vi "Shock&Dyanamics Laboratory - DROPBEAR_June2022_Rev3.vi"() -> ()   [LabVIEW 2019] (continued)
  T49 = cluster{"Voltage Max Ch0":dbl, "Voltage Max Ch 1":dbl, "Voltage Max Ch 2":dbl, "Voltage Max Ch 3":dbl, "Voltage Max Ch 4":dbl, "Voltage Max Ch 5":dbl, "Voltage Max  Ch 6":dbl, "Voltage Max Ch 7":dbl, "Voltage Max Ch 8":dbl, "Voltage Max Ch 9":dbl, "Voltage Max Ch 10":dbl, "Voltage Max Ch 11":dbl, "Voltage Max Ch 12":dbl, "Voltage Max Ch 13":dbl, "Voltage Max Ch 14":dbl, "Voltage Max Ch 15":dbl, "Voltage Max Ch 16":dbl, "Voltage Max Ch 17":dbl, "Voltage Max Ch 18":dbl, "Voltage Max Ch 19":dbl, "Voltage Max Ch 20":dbl, "Voltage Max Ch 21":dbl, "Voltage Max Ch 22":dbl, "Voltage Max Ch 23":dbl, "Voltage Max Ch 24":dbl, "Voltage Max  Ch 7":dbl, "Voltage Max Ch 6":dbl, "Voltage Max Ch 25":dbl, "Voltage Max Ch 26":dbl, "Voltage Max Ch 27":dbl, "Voltage Max Ch 28":dbl, "Voltage Max Ch0 2":dbl}
  T50 = cluster{"Sensitivity 0":dbl, "Sensitivity 1":dbl, "Sensitivity 2":dbl, "Sensitivity 3":dbl, "Sensitivity 4":dbl, "Sensitivity 5":dbl, "Sensitivity 6":dbl, "Sensitivity 7":dbl, "Sensitivity 8":dbl, "Sensitivity 9":dbl, "Sensitivity 10":dbl, "Sensitivity 11":dbl, "Sensitivity 12":dbl, "Sensitivity 13":dbl, "Sensitivity 14":dbl, "Sensitivity 15":dbl, "Sensitivity 16":dbl, "Sensitivity 17":dbl, "Sensitivity 18":dbl, "Sensitivity 19":dbl, "Sensitivity 20":dbl, "Sensitivity 21":dbl, "Sensitivity 22":dbl, "Sensitivity 23":dbl, "Sensitivity 24":dbl, "Sensitivity 25":dbl, "Sensitivity 26":dbl, "Sensitivity 27":dbl, "Sensitivity 28":dbl, "Sensitivity 29":dbl, "Sensitivity 30":dbl, "Sensitivity 31":dbl}
  T51 = cluster{"Sens Fac 0":enum16{"uV/MU", "mV/MU", "V/MU"}, "Sens Fac 1":enum16{"uV/MU", "mV/MU", "V/MU"}, "Sens Fac 2":enum16{"uV/MU", "mV/MU", "V/MU"}, "Sens Fac 3":enum16{"uV/MU", "mV/MU", "V/MU"}, "Sens Fac 4":enum16{"uV/MU", "mV/MU", "V/MU"}, "Sens Fac 5":enum16{"uV/MU", "mV/MU", "V/MU"}, "Sens Fac 6":enum16{"uV/MU", "mV/MU", "V/MU"}, "Sens Fac 7":enum16{"uV/MU", "mV/MU", "V/MU"}, "Sens Fac 8":enum16{"uV/MU", "mV/MU", "V/MU"}, "Sens Fac 9":enum16{"uV/MU", "mV/MU", "V/MU"}, "Sens Fac 10":enum16{"uV/MU", "mV/MU", "V/MU"}, "Sens Fac 11":enum16{"uV/MU", "mV/MU", "V/MU"}, "Sens Fac 12":enum16{"uV/MU", "mV/MU", "V/MU"}, "Sens Fac 13":enum16{"uV/MU", "mV/MU", "V/MU"}, "Sens Fac 14":enum16{"uV/MU", "mV/MU", "V/MU"}, "Sens Fac 15":enum16{"uV/MU", "mV/MU", "V/MU"}, "Sens Fac 16":enum16{"uV/MU", "mV/MU", "V/MU"}, "Sens Fac 17":enum16{"uV/MU", "mV/MU", "V/MU"}, "Sens Fac 18":enum16{"uV/MU", "mV/MU", "V/MU"}, "Sens Fac 19":enum16{"uV/MU", "mV/MU", "V/MU"}, "Sens Fac 20":enum16{"uV/MU", "mV/MU", "V/MU"}, "Sens Fac 21":enum16{"uV/MU", "mV/MU", "V/MU"}, "Sens Fac 22":enum16{"uV/MU", "mV/MU", "V/MU"}, "Sens Fac 23":enum16{"uV/MU", "mV/MU", "V/MU"}, "Sens Fac 24":enum16{"uV/MU", "mV/MU", "V/MU"}, "Sens Fac 25":enum16{"uV/MU", "mV/MU", "V/MU"}, "Sens Fac 26":enum16{"uV/MU", "mV/MU", "V/MU"}, "Sens Fac 27":enum16{"uV/MU", "mV/MU", "V/MU"}, "Sens Fac 28":enum16{"uV/MU", "mV/MU", "V/MU"}, "Sens Fac 29":enum16{"uV/MU", "mV/MU", "V/MU"}, "Sens Fac 30":enum16{"uV/MU", "mV/MU", "V/MU"}, "Sens Fac 31":enum16{"uV/MU", "mV/MU", "V/MU"}}
  T52 = cluster{"SG Pair 0":bool, "SG Pair 1":bool, "SG Pair 2":bool, "SG Pair 3":bool, "SG Pair 4":bool, "SG Pair 5":bool, "SG Pair 6":bool, "SG Pair 7":bool, "SG Pair 8":bool, "SG Pair 9":bool, "SG Pair 10":bool, "SG Pair 11":bool, "SG Pair 12":bool, "SG Pair 13":bool, "SG Pair 14":bool, "SG Pair 15":bool, "SG Pair 16":bool, "SG Pair 17":bool, "SG Pair 18":bool, "SG Pair 19":bool, "SG Pair 20":bool, "SG Pair 21":bool, "SG Pair 22":bool, "SG Pair 23":bool, "SG Pair 24":bool, "SG Pair 25":bool, "SG Pair 26":bool, "SG Pair 27":bool, "SG Pair 28":bool, "SG Pair 29":bool, "SG Pair 30":bool, "SG Pair 31":bool}
  T53 = cluster{"SG Pair Ch 0":enum16{"", "Ch 1", "Ch 2", "Ch 3", "Ch 4", "Ch 5", "Ch 6", "Ch 7", "Ch 8", "Ch 9", "Ch 10", "Ch 11", "Ch 12", "Ch 13", "Ch 14", "Ch 15", "Ch 16", "Ch 17", "Ch 18", "Ch 19", "Ch 20", "Ch 21", "Ch 22", "Ch 23", "Ch 24", "Ch 25", "Ch 26", "Ch 27", "Ch 28", "Ch 29", "Ch 30", "Ch 31", "Paired", "Unpaired"}, "SG Pair Ch 1":enum16{"Ch 0", "", "Ch 2", "Ch 3", "Ch 4", "Ch 5", "Ch 6", "Ch 7", "Ch 8", "Ch 9", "Ch 10", "Ch 11", "Ch 12", "Ch 13", "Ch 14", "Ch 15", "Ch 16", "Ch 17", "Ch 18", "Ch 19", "Ch 20", "Ch 21", "Ch 22", "Ch 23", "Ch 24", "Ch 25", "Ch 26", "Ch 27", "Ch 28", "Ch 29", "Ch 30", "Ch 31", "Paired", "Unpaired"}, "SG Pair Ch 2":enum16{"Ch0", "Ch 1", "", "Ch 3", "Ch 4", "Ch 5", "Ch 6", "Ch 7", "Ch 8", "Ch 9", "Ch 10", "Ch 11", "Ch 12", "Ch 13", "Ch 14", "Ch 15", "Ch 16", "Ch 17", "Ch 18", "Ch 19", "Ch 20", "Ch 21", "Ch 22", "Ch 23", "Ch 24", "Ch 25", "Ch 26", "Ch 27", "Ch 28", "Ch 29", "Ch 30", "Ch 31", "Paired", "Unpaired"}, "SG Pair Ch 3":enum16{"Ch 0", "Ch 1", "Ch 2", "", "Ch 4", "Ch 5", "Ch 6", "Ch 7", "Ch 8", "Ch 9", "Ch 10", "Ch 11", "Ch 12", "Ch 13", "Ch 14", "Ch 15", "Ch 16", "Ch 17", "Ch 18", "Ch 19", "Ch 20", "Ch 21", "Ch 22", "Ch 23", "Ch 24", "Ch 25", "Ch 26", "Ch 27", "Ch 28", "Ch 29", "Ch 30", "Ch 31", "Paired", "Unpaired"}, "SG Pair Ch 4":enum16{"Ch 0", "Ch 1", "Ch 2", "Ch 3", "", "Ch 5", "Ch 6", "Ch 7", "Ch 8", "Ch 9", "Ch 10", "Ch 11", "Ch 12", "Ch 13", "Ch 14", "Ch 15", "Ch 16", "Ch 17", "Ch 18", "Ch 19", "Ch 20", "Ch 21", "Ch 22", "Ch 23", "Ch 24", "Ch 25", "Ch 26", "Ch 27", "Ch 28", "Ch 29", "Ch 30", "Ch 31", "Paired", "Unpaired"}, "SG Pair Ch 5":enum16{"Ch 0", "Ch 1", "Ch 2", "Ch 3", "Ch 4", "", "Ch 6", "Ch 7", "Ch 8", "Ch 9", "Ch 10", "Ch 11", "Ch 12", "Ch 13", "Ch 14", "Ch 15", "Ch 16", "Ch 17", "Ch 18", "Ch 19", "Ch 20", "Ch 21", "Ch 22", "Ch 23", "Ch 24", "Ch 25", "Ch 26", "Ch 27", "Ch 28", "Ch 29", "Ch 30", "Ch 31", "Paired", "Unpaired"}, "SG Pair Ch 6":enum16{"Ch 0", "Ch 1", "Ch 2", "Ch 3", "Ch 4", "Ch 5", "", "Ch 7", "Ch 8", "Ch 9", "Ch 10", "Ch 11", "Ch 12", "Ch 13", "Ch 14", "Ch 15", "Ch 16", "Ch 17", "Ch 18", "Ch 19", "Ch 20", "Ch 21", "Ch 22", "Ch 23", "Ch 24", "Ch 25", "Ch 26", "Ch 27", "Ch 28", "Ch 29", "Ch 30", "Ch 31", "Paired", "Unpaired"}, "SG Pair Ch 7":enum16{"Ch 0", "Ch 1", "Ch 2", "Ch 3", "Ch 4", "Ch 5", "Ch 6", "", "Ch 8", "Ch 9", "Ch 10", "Ch 11", "Ch 12", "Ch 13", "Ch 14", "Ch 15", "Ch 16", "Ch 17", "Ch 18", "Ch 19", "Ch 20", "Ch 21", "Ch 22", "Ch 23", "Ch 24", "Ch 25", "Ch 26", "Ch 27", "Ch 28", "Ch 29", "Ch 30", "Ch 31", "Paired", "Unpaired"}, "SG Pair Ch 8":enum16{"Ch 0", "Ch 1", "Ch 2", "Ch 3", "Ch 4", "Ch 5", "Ch 6", "Ch 7", "", "Ch 9", "Ch 10", "Ch 11", "Ch 12", "Ch 13", "Ch 14", "Ch 15", "Ch 16", "Ch 17", "Ch 18", "Ch 19", "Ch 20", "Ch 21", "Ch 22", "Ch 23", "Ch 24", "Ch 25", "Ch 26", "Ch 27", "Ch 28", "Ch 29", "Ch 30", "Ch 31", "Paired", "Unpaired"}, "SG Pair Ch 9":enum16{"Ch 0", "Ch 1", "Ch 2", "Ch 3", "Ch 4", "Ch 5", "Ch 6", "Ch 7", "Ch 8", "", "Ch 10", "Ch 11", "Ch 12", "Ch 13", "Ch 14", "Ch 15", "Ch 16", "Ch 17", "Ch 18", "Ch 19", "Ch 20", "Ch 21", "Ch 22", "Ch 23", "Ch 24", "Ch 25", "Ch 26", "Ch 27", "Ch 28", "Ch 29", "Ch 30", "Ch 31", "Paired", "Unpaired"}, "SG Pair Ch 10":enum16{"Ch 0", "Ch 1", "Ch 2", "Ch 3", "Ch 4", "Ch 5", "Ch 6", "Ch 7", "Ch 8", "Ch 9", "", "Ch 11", "Ch 12", "Ch 13", "Ch 14", "Ch 15", "Ch 16", "Ch 17", "Ch 18", "Ch 19", "Ch 20", "Ch 21", "Ch 22", "Ch 23", "Ch 24", "Ch 25", "Ch 26", "Ch 27", "Ch 28", "Ch 29", "Ch 30", "Ch 31", "Paired", "Unpaired"}, "SG Pair Ch 11":enum16{"Ch 0", "Ch 1", "Ch 2", "Ch 3", "Ch 4", "Ch 5", "Ch 6", "Ch 7", "Ch 8", "Ch 9", "Ch 10", "", "Ch 12", "Ch 13", "Ch 14", "Ch 15", "Ch 16", "Ch 17", "Ch 18", "Ch 19", "Ch 20", "Ch 21", "Ch 22", "Ch 23", "Ch 24", "Ch 25", "Ch 26", "Ch 27", "Ch 28", "Ch 29", "Ch 30", "Ch 31", "Paired", "Unpaired"}, "SG Pair Ch 12":enum16{"Ch 0", "Ch 1", "Ch 2", "Ch 3", "Ch 4", "Ch 5", "Ch 6", "Ch 7", "Ch 8", "Ch 9", "Ch 10", "Ch 11", "", "Ch 13", "Ch 14", "Ch 15", "Ch 16", "Ch 17", "Ch 18", "Ch 19", "Ch 20", "Ch 21", "Ch 22", "Ch 23", "Ch 24", "Ch 25", "Ch 26", "Ch 27", "Ch 28", "Ch 29", "Ch 30", "Ch 31", "Paired", "Unpaired"}, "SG Pair Ch 13":enum16{"Ch 0", "Ch 1", "Ch 2", "Ch 3", "Ch 4", "Ch 5", "Ch 6", "Ch 7", "Ch 8", "Ch 9", "Ch 10", "Ch 11", "Ch 12", "", "Ch 14", "Ch 15", "Ch 16", "Ch 17", "Ch 18", "Ch 19", "Ch 20", "Ch 21", "Ch 22", "Ch 23", "Ch 24", "Ch 25", "Ch 26", "Ch 27", "Ch 28", "Ch 29", "Ch 30", "Ch 31", "Paired", "Unpaired"}, "SG Pair Ch 14":enum16{"Ch 0", "Ch 1", "Ch 2", "Ch 3", "Ch 4", "Ch 5", "Ch 6", "Ch 7", "Ch 8", "Ch 9", "Ch 10", "Ch 11", "Ch 12", "Ch 13", "", "Ch 15", "Ch 16", "Ch 17", "Ch 18", "Ch 19", "Ch 20", "Ch 21", "Ch 22", "Ch 23", "Ch 24", "Ch 25", "Ch 26", "Ch 27", "Ch 28", "Ch 29", "Ch 30", "Ch 31", "Paired", "Unpaired"}, "SG Pair Ch 15":enum16{"Ch 0", "Ch 1", "Ch 2", "Ch 3", "Ch 4", "Ch 5", "Ch 6", "Ch 7", "Ch 8", "Ch 9", "Ch 10", "Ch 11", "Ch 12", "Ch 13", "Ch 14", "", "Ch 16", "Ch 17", "Ch 18", "Ch 19", "Ch 20", "Ch 21", "Ch 22", "Ch 23", "Ch 24", "Ch 25", "Ch 26", "Ch 27", "Ch 28", "Ch 29", "Ch 30", "Ch 31", "Paired", "Unpaired"}, "SG Pair Ch 16":enum16{"Ch 0", "Ch 1", "Ch 2", "Ch 3", "Ch 4", "Ch 5", "Ch 6", "Ch 7", "Ch 8", "Ch 9", "Ch 10", "Ch 11", "Ch 12", "Ch 13", "Ch 14", "Ch 15", "", "Ch 17", "Ch 18", "Ch 19", "Ch 20", "Ch 21", "Ch 22", "Ch 23", "Ch 24", "Ch 25", "Ch 26", "Ch 27", "Ch 28", "Ch 29", "Ch 30", "Ch 31", "Paired", "Unpaired"}, "SG Pair Ch 17":enum16{"Ch 0", "Ch 1", "Ch 2", "Ch 3", "Ch 4", "Ch 5", "Ch 6", "Ch 7", "Ch 8", "Ch 9", "Ch 10", "Ch 11", "Ch 12", "Ch 13", "Ch 14", "Ch 15", "Ch 16", "", "Ch 18", "Ch 19", "Ch 20", "Ch 21", "Ch 22", "Ch 23", "Ch 24", "Ch 25", "Ch 26", "Ch 27", "Ch 28", "Ch 29", "Ch 30", "Ch 31", "Paired", "Unpaired"}, "SG Pair Ch 18":enum16{"Ch 0", "Ch 1", "Ch 2", "Ch 3", "Ch 4", "Ch 5", "Ch 6", "Ch 7", "Ch 8", "Ch 9", "Ch 10", "Ch 11", "Ch 12", "Ch 13", "Ch 14", "Ch 15", "Ch 16", "Ch 17", "", "Ch 19", "Ch 20", "Ch 21", "Ch 22", "Ch 23", "Ch 24", "Ch 25", "Ch 26", "Ch 27", "Ch 28", "Ch 29", "Ch 30", "Ch 31", "Paired", "Unpaired"}, "SG Pair Ch 19":enum16{"Ch 0", "Ch 1", "Ch 2", "Ch 3", "Ch 4", "Ch 5", "Ch 6", "Ch 7", "Ch 8", "Ch 9", "Ch 10", "Ch 11", "Ch 12", "Ch 13", "Ch 14", "Ch 15", "Ch 16", "Ch 17", "Ch 18", "", "Ch 20", "Ch 21", "Ch 22", "Ch 23", "Ch 24", "Ch 25", "Ch 26", "Ch 27", "Ch 28", "Ch 29", "Ch 30", "Ch 31", "Paired", "Unpaired"}, "SG Pair Ch 20":enum16{"Ch 0", "Ch 1", "Ch 2", "Ch 3", "Ch 4", "Ch 5", "Ch 6", "Ch 7", "Ch 8", "Ch 9", "Ch 10", "Ch 11", "Ch 12", "Ch 13", "Ch 14", "Ch 15", "Ch 16", "Ch 17", "Ch 18", "Ch 19", "", "Ch 21", "Ch 22", "Ch 23", "Ch 24", "Ch 25", "Ch 26", "Ch 27", "Ch 28", "Ch 29", "Ch 30", "Ch 31", "Paired", "Unpaired"}, "SG Pair Ch 21":enum16{"Ch 0", "Ch 1", "Ch 2", "Ch 3", "Ch 4", "Ch 5", "Ch 6", "Ch 7", "Ch 8", "Ch 9", "Ch 10", "Ch 11", "Ch 12", "Ch 13", "Ch 14", "Ch 15", "Ch 16", "Ch 17", "Ch 18", "Ch 19", "Ch 20", "", "Ch 22", "Ch 23", "Ch 24", "Ch 25", "Ch 26", "Ch 27", "Ch 28", "Ch 29", "Ch 30", "Ch 31", "Paired", "Unpaired"}, "SG Pair Ch 22":enum16{"Ch 0", "Ch 1", "Ch 2", "Ch 3", "Ch 4", "Ch 5", "Ch 6", "Ch 7", "Ch 8", "Ch 9", "Ch 10", "Ch 11", "Ch 12", "Ch 13", "Ch 14", "Ch 15", "Ch 16", "Ch 17", "Ch 18", "Ch 19", "Ch 20", "Ch 21", "", "Ch 23", "Ch 24", "Ch 25", "Ch 26", "Ch 27", "Ch 28", "Ch 29", "Ch 30", "Ch 31", "Paired", "Unpaired"}, "SG Pair Ch 23":enum16{"Ch 0", "Ch 1", "Ch 2", "Ch 3", "Ch 4", "Ch 5", "Ch 6", "Ch 7", "Ch 8", "Ch 9", "Ch 10", "Ch 11", "Ch 12", "Ch 13", "Ch 14", "Ch 15", "Ch 16", "Ch 17", "Ch 18", "Ch 19", "Ch 20", "Ch 21", "Ch 22", "", "Ch 24", "Ch 25", "Ch 26", "Ch 27", "Ch 28", "Ch 29", "Ch 30", "Ch 31", "Paired", "Unpaired"}, "SG Pair Ch 24":enum16{"Ch 0", "Ch 1", "Ch 2", "Ch 3", "Ch 4", "Ch 5", "Ch 6", "Ch 7", "Ch 8", "Ch 9", "Ch 10", "Ch 11", "Ch 12", "Ch 13", "Ch 14", "Ch 15", "Ch 16", "Ch 17", "Ch 18", "Ch 19", "Ch 20", "Ch 21", "Ch 22", "Ch 23", "", "Ch 25", "Ch 26", "Ch 27", "Ch 28", "Ch 29", "Ch 30", "Ch 31", "Paired", "Unpaired"}, "SG Pair Ch 25":enum16{"Ch 0", "Ch 1", "Ch 2", "Ch 3", "Ch 4", "Ch 5", "Ch 6", "Ch 7", "Ch 8", "Ch 9", "Ch 10", "Ch 11", "Ch 12", "Ch 13", "Ch 14", "Ch 15", "Ch 16", "Ch 17", "Ch 18", "Ch 19", "Ch 20", "Ch 21", "Ch 22", "Ch 23", "Ch 24", "", "Ch 26", "Ch 27", "Ch 28", "Ch 29", "Ch 30", "Ch 31", "Paired", "Unpaired"}, "SG Pair Ch 26":enum16{"Ch 0", "Ch 1", "Ch 2", "Ch 3", "Ch 4", "Ch 5", "Ch 6", "Ch 7", "Ch 8", "Ch 9", "Ch 10", "Ch 11", "Ch 12", "Ch 13", "Ch 14", "Ch 15", "Ch 16", "Ch 17", "Ch 18", "Ch 19", "Ch 20", "Ch 21", "Ch 22", "Ch 23", "Ch 24", "Ch 25", "", "Ch 27", "Ch 28", "Ch 29", "Ch 30", "Ch 31", "Paired", "Unpaired"}, "SG Pair Ch 27":enum16{"Ch 0", "Ch 1", "Ch 2", "Ch 3", "Ch 4", "Ch 5", "Ch 6", "Ch 7", "Ch 8", "Ch 9", "Ch 10", "Ch 11", "Ch 12", "Ch 13", "Ch 14", "Ch 15", "Ch 16", "Ch 17", "Ch 18", "Ch 19", "Ch 20", "Ch 21", "Ch 22", "Ch 23", "Ch 24", "Ch 25", "Ch 26", "", "Ch 28", "Ch 29", "Ch 30", "Ch 31", "Paired", "Unpaired"}, "SG Pair Ch 28":enum16{"Ch 0", "Ch 1", "Ch 2", "Ch 3", "Ch 4", "Ch 5", "Ch 6", "Ch 7", "Ch 8", "Ch 9", "Ch 10", "Ch 11", "Ch 12", "Ch 13", "Ch 14", "Ch 15", "Ch 16", "Ch 17", "Ch 18", "Ch 19", "Ch 20", "Ch 21", "Ch 22", "Ch 23", "Ch 24", "Ch 25", "Ch 26", "Ch 27", "", "Ch 29", "Ch 30", "Ch 31", "Paired", "Unpaired"}, "SG Pair Ch 29":enum16{"Ch 0", "Ch 1", "Ch 2", "Ch 3", "Ch 4", "Ch 5", "Ch 6", "Ch 7", "Ch 8", "Ch 9", "Ch 10", "Ch 11", "Ch 12", "Ch 13", "Ch 14", "Ch 15", "Ch 16", "Ch 17", "Ch 18", "Ch 19", "Ch 20", "Ch 21", "Ch 22", "Ch 23", "Ch 24", "Ch 25", "Ch 26", "Ch 27", "Ch 28", "", "Ch 30", "Ch 31", "Paired", "Unpaired"}, "SG Pair Ch 30":enum16{"Ch 0", "Ch 1", "Ch 2", "Ch 3", "Ch 4", "Ch 5", "Ch 6", "Ch 7", "Ch 8", "Ch 9", "Ch 10", "Ch 11", "Ch 12", "Ch 13", "Ch 14", "Ch 15", "Ch 16", "Ch 17", "Ch 18", "Ch 19", "Ch 20", "Ch 21", "Ch 22", "Ch 23", "Ch 24", "Ch 25", "Ch 26", "Ch 27", "Ch 28", "Ch 29", "", "Ch 31", "Paired", "Unpaired"}, "SG Pair Ch 31":enum16{"Ch 0", "Ch 1", "Ch 2", "Ch 3", "Ch 4", "Ch 5", "Ch 6", "Ch 7", "Ch 8", "Ch 9", "Ch 10", "Ch 11", "Ch 12", "Ch 13", "Ch 14", "Ch 15", "Ch 16", "Ch 17", "Ch 18", "Ch 19", "Ch 20", "Ch 21", "Ch 22", "Ch 23", "Ch 24", "Ch 25", "Ch 26", "Ch 27", "Ch 28", "Ch 29", "Ch 30", "", "Paired", "Unpaired"}}
  T54 = cluster{"PF Condition 0":bool, "PF Condition 1":bool, "PF Condition 2":bool, "PF Condition 3":bool, "PF Condition 4":bool, "PF Condition 5":bool, "PF Condition 6":bool, "PF Condition 7":bool, "PF Condition 8":bool, "PF Condition 9":bool, "PF Condition 10":bool, "PF Condition 11":bool, "PF Condition 12":bool, "PF Condition 13":bool, "PF Condition 14":bool, "PF Condition 15":bool, "PF Condition 16":bool, "PF Condition 17":bool, "PF Condition 18":bool, "PF Condition 19":bool, "PF Condition 20":bool, "PF Condition 21":bool, "PF Condition 22":bool, "PF Condition 23":bool, "PF Condition 24":bool, "PF Condition 25":bool, "PF Condition 26":bool, "PF Condition 27":bool, "PF Condition 28":bool, "PF Condition 29":bool, "PF Condition 30":bool, "PF Condition 31":bool}
  T55 = cluster{"PF Info":string, "PF Info":string, "PF Info":string, "PF Info":string, "PF Info":string, "PF Info":string, "PF Info":string, "PF Info":string, "PF Info":string, "PF Info":string, "PF Info":string, "PF Info":string, "PF Info":string, "PF Info":string, "PF Info":string, "PF Info":string, "PF Info 2":string, "PF Info 3":string, "PF Info 4":string, "PF Info 5":string, "PF Info 6":string, "PF Info 7":string, "PF Info 8":string, "PF Info 9":string, "PF Info 10":string, "PF Info 11":string, "PF Info 12":string, "PF Info 13":string, "PF Info 14":string, "PF Info 15":string, "PF Info 16":string, "PF Info 17":string}
  T56 = cluster{"Value":cluster{cluster{bool, "Enable Ch 1":bool, "Enable Ch 2":bool, "Enable Ch 3":bool, "Enable Ch 4":bool, "Enable Ch 5":bool, "Enable Ch 6":bool, "Enable Ch 7":bool, "Enable Ch 8":bool, "Enable Ch 9":bool, "Enable Ch 10":bool, "Enable Ch 11":bool, "Enable Ch 12":bool, "Enable Ch 13":bool, "Enable Ch 14":bool, "Enable Ch 15":bool, "Enable Ch 16":bool, "Enable Ch 17":bool, "Enable Ch 18":bool, "Enable Ch 19":bool, "Enable Ch 20":bool, "Enable Ch 21":bool, "Enable Ch 22":bool, "Enable Ch 23":bool, "Enable Ch 24":bool, "Enable Ch 25":bool, "Enable Ch 26":bool, "Enable Ch 27":bool, "Enable Ch 28":bool, "Enable Ch 29":bool, "Enable Ch 30":bool, "Enable Ch 31":bool}, cluster{"Name (Laser Gate)":string, "Name Ch 1":string, "Name Ch 2":string, "Name Ch 3":string, "Name Ch 4":string, "Name Ch 5":string, "Name Ch 6":string, "Name Ch 7":string, "Name Ch 8":string, "Name Ch 9":string, "Name Ch 10":string, "Name Ch 11":string, "Name Ch 12":string, "Name Ch 13":string, "Name Ch 14":string, "Name Ch 15":string, "Name Ch 16":string, "Name Ch 17":string, "Name Ch 18":string, "Name Ch 19":string, "Name Ch 20":string, "Name Ch 21":string, "Name Ch 22":string, "Name Ch 23":string, "Name Ch 24":string, "Name Ch 25":string, "Name Ch 26":string, "Name Ch 27":string, "Name Ch 28":string, "Name Ch 29":string, "Name Ch 30":string, "Name Ch 31":string}, cluster{"Physical Channels Ch 0":tag, "Physical Channel Ch 1":tag, "Physical Channel Ch 2":tag, "Physical Channels Ch 3":tag, "Physical Channel Ch 4":tag, "Physical Channel Ch 5":tag, "Physical Channels Ch 6":tag, "Physical Channel Ch 7":tag, "Physical Channel Ch 8":tag, "Physical Channel Ch 9":tag, "Physical Channel Ch 10":tag, "Physical Channel Ch 11":tag, "Physical Channel Ch 12":tag, "Physical Channel Ch 13":tag, "Physical Channel Ch 14":tag, "Physical Channel Ch 15":tag, "Physical Channel Ch 16":tag, "Physical Channel Ch 17":tag, "Physical Channel Ch 18":tag, "Physical Channel Ch 19":tag, "Physical Channel Ch 20":tag, "Physical Channel Ch 21":tag, "Physical Channel Ch 22":tag, "Physical Channel Ch 23":tag, "Physical Channel Ch 24":tag, "Physical Channel Ch 25":tag, "Physical Channel Ch 26":tag, "Physical Channel Ch 27":tag, "Physical Channel Ch 28":tag, "Physical Channel Ch 29":tag, "Physical Channel Ch 30":tag, "Physical Channel Ch 31":tag}, cluster{"Voltage Min Ch 0":dbl, "Voltage Min Ch 1":dbl, "Voltage Min Ch 2":dbl, "Voltage Min Ch 3":dbl, "Voltage Min Ch 4":dbl, "Voltage Min Ch 5":dbl, "Voltage Min Ch 6":dbl, "Voltage Min Ch 7":dbl, "Voltage Min Ch 8":dbl, "Voltage Min Ch 9":dbl, "Voltage Min Ch 10":dbl, "Voltage Min Ch 11":dbl, "Voltage Min Ch 12":dbl, "Voltage Min Ch 13":dbl, "Voltage Min Ch 14":dbl, "Voltage Min Ch 15":dbl, "Voltage Min Ch 16":dbl, "Voltage Min Ch 17":dbl, "Voltage Min Ch 18":dbl, "Voltage Min Ch 19":dbl, "Voltage Min Ch 20":dbl, "Voltage Min Ch 21":dbl, "Voltage Min Ch 22":dbl, "Voltage Min Ch 23":dbl, "Voltage Min Ch 24":dbl, "Voltage Min Ch 25":dbl, "Voltage Min Ch 26":dbl, "Voltage Min Ch 27":dbl, "Voltage Min Ch 28":dbl, "Voltage Min Ch 29":dbl, "Voltage Min Ch 30":dbl, "Voltage Min Ch 31":dbl}, cluster{"Voltage Max Ch 0":dbl, "Voltage Max Ch 1":dbl, "Voltage Max Ch 2":dbl, "Voltage Max Ch 3":dbl, "Voltage Max Ch 4":dbl, "Voltage Max Ch 5":dbl, "Voltage Max  Ch 6":dbl, "Voltage Max Ch 7":dbl, "Voltage Max Ch 8":dbl, "Voltage Max Ch 9":dbl, "Voltage Max Ch 10":dbl, "Voltage Max Ch 11":dbl, "Voltage Max Ch 12":dbl, "Voltage Max Ch 13":dbl, "Voltage Max Ch 14":dbl, "Voltage Max Ch 15":dbl, "Voltage Max Ch 16":dbl, "Voltage Max Ch 17":dbl, "Voltage Max Ch 18":dbl, "Voltage Max Ch 19":dbl, "Voltage Max Ch 20":dbl, "Voltage Max Ch 21":dbl, "Voltage Max Ch 22":dbl, "Voltage Max Ch 23":dbl, "Voltage Max Ch 24":dbl, "Voltage Max Ch 25":dbl, "Voltage Max Ch 26":dbl, "Voltage Max Ch 27":dbl, "Voltage Max Ch 28":dbl, "Voltage Max Ch 29":dbl, "Voltage Max Ch 30":dbl, "Voltage Max Ch 31":dbl}, cluster{"Sensitivity 0":dbl, "Sensitivity 1":dbl, "Sensitivity 2":dbl, "Sensitivity 3":dbl, "Sensitivity 4":dbl, "Sensitivity 5":dbl, "Sensitivity 6":dbl, "Sensitivity 7":dbl, "Sensitivity 8":dbl, "Sensitivity 9":dbl, "Sensitivity 10":dbl, "Sensitivity 11":dbl, "Sensitivity 12":dbl, "Sensitivity 13":dbl, "Sensitivity 14":dbl, "Sensitivity 15":dbl, "Sensitivity 16":dbl, "Sensitivity 17":dbl, "Sensitivity 18":dbl, "Sensitivity 19":dbl, "Sensitivity 20":dbl, "Sensitivity 21":dbl, "Sensitivity 22":dbl, "Sensitivity 23":dbl, "Sensitivity 24":dbl, "Sensitivity 25":dbl, "Sensitivity 26":dbl, "Sensitivity 27":dbl, "Sensitivity 28":dbl, "Sensitivity 29":dbl, "Sensitivity 30":dbl, "Sensitivity 31":dbl}, cluster{"Sens Fac 0":enum16{"uV/MU", "mV/MU", "V/MU"}, "Sens Fac 1":enum16{"uV/MU", "mV/MU", "V/MU"}, "Sens Fac 2":enum16{"uV/MU", "mV/MU", "V/MU"}, "Sens Fac 3":enum16{"uV/MU", "mV/MU", "V/MU"}, "Sens Fac 4":enum16{"uV/MU", "mV/MU", "V/MU"}, "Sens Fac 5":enum16{"uV/MU", "mV/MU", "V/MU"}, "Sens Fac 6":enum16{"uV/MU", "mV/MU", "V/MU"}, "Sens Fac 7":enum16{"uV/MU", "mV/MU", "V/MU"}, "Sens Fac 8":enum16{"uV/MU", "mV/MU", "V/MU"}, "Sens Fac 9":enum16{"uV/MU", "mV/MU", "V/MU"}, "Sens Fac 10":enum16{"uV/MU", "mV/MU", "V/MU"}, "Sens Fac 11":enum16{"uV/MU", "mV/MU", "V/MU"}, "Sens Fac 12":enum16{"uV/MU", "mV/MU", "V/MU"}, "Sens Fac 13":enum16{"uV/MU", "mV/MU", "V/MU"}, "Sens Fac 14":enum16{"uV/MU", "mV/MU", "V/MU"}, "Sens Fac 15":enum16{"uV/MU", "mV/MU", "V/MU"}, "Sens Fac 16":enum16{"uV/MU", "mV/MU", "V/MU"}, "Sens Fac 17":enum16{"uV/MU", "mV/MU", "V/MU"}, "Sens Fac 18":enum16{"uV/MU", "mV/MU", "V/MU"}, "Sens Fac 19":enum16{"uV/MU", "mV/MU", "V/MU"}, "Sens Fac 20":enum16{"uV/MU", "mV/MU", "V/MU"}, "Sens Fac 21":enum16{"uV/MU", "mV/MU", "V/MU"}, "Sens Fac 22":enum16{"uV/MU", "mV/MU", "V/MU"}, "Sens Fac 23":enum16{"uV/MU", "mV/MU", "V/MU"}, "Sens Fac 24":enum16{"uV/MU", "mV/MU", "V/MU"}, "Sens Fac 25":enum16{"uV/MU", "mV/MU", "V/MU"}, "Sens Fac 26":enum16{"uV/MU", "mV/MU", "V/MU"}, "Sens Fac 27":enum16{"uV/MU", "mV/MU", "V/MU"}, "Sens Fac 28":enum16{"uV/MU", "mV/MU", "V/MU"}, "Sens Fac 29":enum16{"uV/MU", "mV/MU", "V/MU"}, "Sens Fac 30":enum16{"uV/MU", "mV/MU", "V/MU"}, "Sens Fac 31":enum16{"uV/MU", "mV/MU", "V/MU"}}, cluster{"Signal Type 0":enum16{"Acceleration", "Velocity", "Strain", "Voltage"}, "Signal Type 1":enum16{"Acceleration", "Velocity", "Strain", "Voltage"}, "Signal Type 2":enum16{"Acceleration", "Velocity", "Strain", "Voltage"}, "Signal Type 3":enum16{"Acceleration", "Velocity", "Strain", "Voltage"}, "Signal Type 4":enum16{"Acceleration", "Velocity", "Strain", "Voltage"}, "Signal Type 5":enum16{"Acceleration", "Velocity", "Strain", "Voltage"}, "Signal Type 6":enum16{"Acceleration", "Velocity", "Strain", "Voltage"}, "Signal Type 7":enum16{"Acceleration", "Velocity", "Strain", "Voltage"}, "Signal Type 8":enum16{"Acceleration", "Velocity", "Strain", "Voltage"}, "Signal Type 9":enum16{"Acceleration", "Velocity", "Strain", "Voltage"}, "Signal Type 10":enum16{"Acceleration", "Velocity", "Strain", "Voltage"}, "Signal Type 11":enum16{"Acceleration", "Velocity", "Strain", "Voltage"}, "Signal Type 12":enum16{"Acceleration", "Velocity", "Strain", "Voltage"}, "Signal Type 13":enum16{"Acceleration", "Velocity", "Strain", "Voltage"}, "Signal Type 14":enum16{"Acceleration", "Velocity", "Strain", "Voltage"}, "Signal Type 15":enum16{"Acceleration", "Velocity", "Strain", "Voltage"}, "Signal Type 16":enum16{"Acceleration", "Velocity", "Strain", "Voltage"}, "Signal Type 17":enum16{"Acceleration", "Velocity", "Strain", "Voltage"}, "Signal Type 18":enum16{"Acceleration", "Velocity", "Strain", "Voltage"}, "Signal Type 19":enum16{"Acceleration", "Velocity", "Strain", "Voltage"}, "Signal Type 20":enum16{"Acceleration", "Velocity", "Strain", "Voltage"}, "Signal Type 21":enum16{"Acceleration", "Velocity", "Strain", "Voltage"}, "Signal Type 22":enum16{"Acceleration", "Velocity", "Strain", "Voltage"}, "Signal Type 23":enum16{"Acceleration", "Velocity", "Strain", "Voltage"}, "Signal Type 24":enum16{"Acceleration", "Velocity", "Strain", "Voltage"}, "Signal Type 25":enum16{"Acceleration", "Velocity", "Strain", "Voltage"}, "Signal Type 26":enum16{"Acceleration", "Velocity", "Strain", "Voltage"}, "Signal Type 27":enum16{"Acceleration", "Velocity", "Strain", "Voltage"}, "Signal Type 28":enum16{"Acceleration", "Velocity", "Strain", "Voltage"}, "Signal Type 29":enum16{"Acceleration", "Velocity", "Strain", "Voltage"}, "Signal Type 30":enum16{"Acceleration", "Velocity", "Strain", "Voltage"}, "Signal Type 31":enum16{"Acceleration", "Velocity", "Strain", "Voltage"}}, cluster{"SG Pair 0":bool, "SG Pair 1":bool, "SG Pair 2":bool, "SG Pair 3":bool, "SG Pair 4":bool, "SG Pair 5":bool, "SG Pair 6":bool, "SG Pair 7":bool, "SG Pair 8":bool, "SG Pair 9":bool, "SG Pair 10":bool, "SG Pair 11":bool, "SG Pair 12":bool, "SG Pair 13":bool, "SG Pair 14":bool, "SG Pair 15":bool, "SG Pair 16":bool, "SG Pair 17":bool, "SG Pair 18":bool, "SG Pair 19":bool, "SG Pair 20":bool, "SG Pair 21":bool, "SG Pair 22":bool, "SG Pair 23":bool, "SG Pair 24":bool, "SG Pair 25":bool, "SG Pair 26":bool, "SG Pair 27":bool, "SG Pair 28":bool, "SG Pair 29":bool, "SG Pair 30":bool, "SG Pair 31":bool}, cluster{"SG Pair Ch 0":enum16{"", "Ch 1", "Ch 2", "Ch 3", "Ch 4", "Ch 5", "Ch 6", "Ch 7", "Ch 8", "Ch 9", "Ch 10", "Ch 11", "Ch 12", "Ch 13", "Ch 14", "Ch 15", "Ch 16", "Ch 17", "Ch 18", "Ch 19", "Ch 20", "Ch 21", "Ch 22", "Ch 23", "Ch 24", "Ch 25", "Ch 26", "Ch 27", "Ch 28", "Ch 29", "Ch 30", "Ch 31", "Paired", "Unpaired"}, "SG Pair Ch 1":enum16{"Ch 0", "", "Ch 2", "Ch 3", "Ch 4", "Ch 5", "Ch 6", "Ch 7", "Ch 8", "Ch 9", "Ch 10", "Ch 11", "Ch 12", "Ch 13", "Ch 14", "Ch 15", "Ch 16", "Ch 17", "Ch 18", "Ch 19", "Ch 20", "Ch 21", "Ch 22", "Ch 23", "Ch 24", "Ch 25", "Ch 26", "Ch 27", "Ch 28", "Ch 29", "Ch 30", "Ch 31", "Paired", "Unpaired"}, "SG Pair Ch 2":enum16{"Ch0", "Ch 1", "", "Ch 3", "Ch 4", "Ch 5", "Ch 6", "Ch 7", "Ch 8", "Ch 9", "Ch 10", "Ch 11", "Ch 12", "Ch 13", "Ch 14", "Ch 15", "Ch 16", "Ch 17", "Ch 18", "Ch 19", "Ch 20", "Ch 21", "Ch 22", "Ch 23", "Ch 24", "Ch 25", "Ch 26", "Ch 27", "Ch 28", "Ch 29", "Ch 30", "Ch 31", "Paired", "Unpaired"}, "SG Pair Ch 3":enum16{"Ch 0", "Ch 1", "Ch 2", "", "Ch 4", "Ch 5", "Ch 6", "Ch 7", "Ch 8", "Ch 9", "Ch 10", "Ch 11", "Ch 12", "Ch 13", "Ch 14", "Ch 15", "Ch 16", "Ch 17", "Ch 18", "Ch 19", "Ch 20", "Ch 21", "Ch 22", "Ch 23", "Ch 24", "Ch 25", "Ch 26", "Ch 27", "Ch 28", "Ch 29", "Ch 30", "Ch 31", "Paired", "Unpaired"}, "SG Pair Ch 4":enum16{"Ch 0", "Ch 1", "Ch 2", "Ch 3", "", "Ch 5", "Ch 6", "Ch 7", "Ch 8", "Ch 9", "Ch 10", "Ch 11", "Ch 12", "Ch 13", "Ch 14", "Ch 15", "Ch 16", "Ch 17", "Ch 18", "Ch 19", "Ch 20", "Ch 21", "Ch 22", "Ch 23", "Ch 24", "Ch 25", "Ch 26", "Ch 27", "Ch 28", "Ch 29", "Ch 30", "Ch 31", "Paired", "Unpaired"}, "SG Pair Ch 5":enum16{"Ch 0", "Ch 1", "Ch 2", "Ch 3", "Ch 4", "", "Ch 6", "Ch 7", "Ch 8", "Ch 9", "Ch 10", "Ch 11", "Ch 12", "Ch 13", "Ch 14", "Ch 15", "Ch 16", "Ch 17", "Ch 18", "Ch 19", "Ch 20", "Ch 21", "Ch 22", "Ch 23", "Ch 24", "Ch 25", "Ch 26", "Ch 27", "Ch 28", "Ch 29", "Ch 30", "Ch 31", "Paired", "Unpaired"}, "SG Pair Ch 6":enum16{"Ch 0", "Ch 1", "Ch 2", "Ch 3", "Ch 4", "Ch 5", "", "Ch 7", "Ch 8", "Ch 9", "Ch 10", "Ch 11", "Ch 12", "Ch 13", "Ch 14", "Ch 15", "Ch 16", "Ch 17", "Ch 18", "Ch 19", "Ch 20", "Ch 21", "Ch 22", "Ch 23", "Ch 24", "Ch 25", "Ch 26", "Ch 27", "Ch 28", "Ch 29", "Ch 30", "Ch 31", "Paired", "Unpaired"}, "SG Pair Ch 7":enum16{"Ch 0", "Ch 1", "Ch 2", "Ch 3", "Ch 4", "Ch 5", "Ch 6", "", "Ch 8", "Ch 9", "Ch 10", "Ch 11", "Ch 12", "Ch 13", "Ch 14", "Ch 15", "Ch 16", "Ch 17", "Ch 18", "Ch 19", "Ch 20", "Ch 21", "Ch 22", "Ch 23", "Ch 24", "Ch 25", "Ch 26", "Ch 27", "Ch 28", "Ch 29", "Ch 30", "Ch 31", "Paired", "Unpaired"}, "SG Pair Ch 8":enum16{"Ch 0", "Ch 1", "Ch 2", "Ch 3", "Ch 4", "Ch 5", "Ch 6", "Ch 7", "", "Ch 9", "Ch 10", "Ch 11", "Ch 12", "Ch 13", "Ch 14", "Ch 15", "Ch 16", "Ch 17", "Ch 18", "Ch 19", "Ch 20", "Ch 21", "Ch 22", "Ch 23", "Ch 24", "Ch 25", "Ch 26", "Ch 27", "Ch 28", "Ch 29", "Ch 30", "Ch 31", "Paired", "Unpaired"}, "SG Pair Ch 9":enum16{"Ch 0", "Ch 1", "Ch 2", "Ch 3", "Ch 4", "Ch 5", "Ch 6", "Ch 7", "Ch 8", "", "Ch 10", "Ch 11", "Ch 12", "Ch 13", "Ch 14", "Ch 15", "Ch 16", "Ch 17", "Ch 18", "Ch 19", "Ch 20", "Ch 21", "Ch 22", "Ch 23", "Ch 24", "Ch 25", "Ch 26", "Ch 27", "Ch 28", "Ch 29", "Ch 30", "Ch 31", "Paired", "Unpaired"}, "SG Pair Ch 10":enum16{"Ch 0", "Ch 1", "Ch 2", "Ch 3", "Ch 4", "Ch 5", "Ch 6", "Ch 7", "Ch 8", "Ch 9", "", "Ch 11", "Ch 12", "Ch 13", "Ch 14", "Ch 15", "Ch 16", "Ch 17", "Ch 18", "Ch 19", "Ch 20", "Ch 21", "Ch 22", "Ch 23", "Ch 24", "Ch 25", "Ch 26", "Ch 27", "Ch 28", "Ch 29", "Ch 30", "Ch 31", "Paired", "Unpaired"}, "SG Pair Ch 11":enum16{"Ch 0", "Ch 1", "Ch 2", "Ch 3", "Ch 4", "Ch 5", "Ch 6", "Ch 7", "Ch 8", "Ch 9", "Ch 10", "", "Ch 12", "Ch 13", "Ch 14", "Ch 15", "Ch 16", "Ch 17", "Ch 18", "Ch 19", "Ch 20", "Ch 21", "Ch 22", "Ch 23", "Ch 24", "Ch 25", "Ch 26", "Ch 27", "Ch 28", "Ch 29", "Ch 30", "Ch 31", "Paired", "Unpaired"}, "SG Pair Ch 12":enum16{"Ch 0", "Ch 1", "Ch 2", "Ch 3", "Ch 4", "Ch 5", "Ch 6", "Ch 7", "Ch 8", "Ch 9", "Ch 10", "Ch 11", "", "Ch 13", "Ch 14", "Ch 15", "Ch 16", "Ch 17", "Ch 18", "Ch 19", "Ch 20", "Ch 21", "Ch 22", "Ch 23", "Ch 24", "Ch 25", "Ch 26", "Ch 27", "Ch 28", "Ch 29", "Ch 30", "Ch 31", "Paired", "Unpaired"}, "SG Pair Ch 13":enum16{"Ch 0", "Ch 1", "Ch 2", "Ch 3", "Ch 4", "Ch 5", "Ch 6", "Ch 7", "Ch 8", "Ch 9", "Ch 10", "Ch 11", "Ch 12", "", "Ch 14", "Ch 15", "Ch 16", "Ch 17", "Ch 18", "Ch 19", "Ch 20", "Ch 21", "Ch 22", "Ch 23", "Ch 24", "Ch 25", "Ch 26", "Ch 27", "Ch 28", "Ch 29", "Ch 30", "Ch 31", "Paired", "Unpaired"}, "SG Pair Ch 14":enum16{"Ch 0", "Ch 1", "Ch 2", "Ch 3", "Ch 4", "Ch 5", "Ch 6", "Ch 7", "Ch 8", "Ch 9", "Ch 10", "Ch 11", "Ch 12", "Ch 13", "", "Ch 15", "Ch 16", "Ch 17", "Ch 18", "Ch 19", "Ch 20", "Ch 21", "Ch 22", "Ch 23", "Ch 24", "Ch 25", "Ch 26", "Ch 27", "Ch 28", "Ch 29", "Ch 30", "Ch 31", "Paired", "Unpaired"}, "SG Pair Ch 15":enum16{"Ch 0", "Ch 1", "Ch 2", "Ch 3", "Ch 4", "Ch 5", "Ch 6", "Ch 7", "Ch 8", "Ch 9", "Ch 10", "Ch 11", "Ch 12", "Ch 13", "Ch 14", "", "Ch 16", "Ch 17", "Ch 18", "Ch 19", "Ch 20", "Ch 21", "Ch 22", "Ch 23", "Ch 24", "Ch 25", "Ch 26", "Ch 27", "Ch 28", "Ch 29", "Ch 30", "Ch 31", "Paired", "Unpaired"}, "SG Pair Ch 16":enum16{"Ch 0", "Ch 1", "Ch 2", "Ch 3", "Ch 4", "Ch 5", "Ch 6", "Ch 7", "Ch 8", "Ch 9", "Ch 10", "Ch 11", "Ch 12", "Ch 13", "Ch 14", "Ch 15", "", "Ch 17", "Ch 18", "Ch 19", "Ch 20", "Ch 21", "Ch 22", "Ch 23", "Ch 24", "Ch 25", "Ch 26", "Ch 27", "Ch 28", "Ch 29", "Ch 30", "Ch 31", "Paired", "Unpaired"}, "SG Pair Ch 17":enum16{"Ch 0", "Ch 1", "Ch 2", "Ch 3", "Ch 4", "Ch 5", "Ch 6", "Ch 7", "Ch 8", "Ch 9", "Ch 10", "Ch 11", "Ch 12", "Ch 13", "Ch 14", "Ch 15", "Ch 16", "", "Ch 18", "Ch 19", "Ch 20", "Ch 21", "Ch 22", "Ch 23", "Ch 24", "Ch 25", "Ch 26", "Ch 27", "Ch 28", "Ch 29", "Ch 30", "Ch 31", "Paired", "Unpaired"}, "SG Pair Ch 18":enum16{"Ch 0", "Ch 1", "Ch 2", "Ch 3", "Ch 4", "Ch 5", "Ch 6", "Ch 7", "Ch 8", "Ch 9", "Ch 10", "Ch 11", "Ch 12", "Ch 13", "Ch 14", "Ch 15", "Ch 16", "Ch 17", "", "Ch 19", "Ch 20", "Ch 21", "Ch 22", "Ch 23", "Ch 24", "Ch 25", "Ch 26", "Ch 27", "Ch 28", "Ch 29", "Ch 30", "Ch 31", "Paired", "Unpaired"}, "SG Pair Ch 19":enum16{"Ch 0", "Ch 1", "Ch 2", "Ch 3", "Ch 4", "Ch 5", "Ch 6", "Ch 7", "Ch 8", "Ch 9", "Ch 10", "Ch 11", "Ch 12", "Ch 13", "Ch 14", "Ch 15", "Ch 16", "Ch 17", "Ch 18", "", "Ch 20", "Ch 21", "Ch 22", "Ch 23", "Ch 24", "Ch 25", "Ch 26", "Ch 27", "Ch 28", "Ch 29", "Ch 30", "Ch 31", "Paired", "Unpaired"}, "SG Pair Ch 20":enum16{"Ch 0", "Ch 1", "Ch 2", "Ch 3", "Ch 4", "Ch 5", "Ch 6", "Ch 7", "Ch 8", "Ch 9", "Ch 10", "Ch 11", "Ch 12", "Ch 13", "Ch 14", "Ch 15", "Ch 16", "Ch 17", "Ch 18", "Ch 19", "", "Ch 21", "Ch 22", "Ch 23", "Ch 24", "Ch 25", "Ch 26", "Ch 27", "Ch 28", "Ch 29", "Ch 30", "Ch 31", "Paired", "Unpaired"}, "SG Pair Ch 21":enum16{"Ch 0", "Ch 1", "Ch 2", "Ch 3", "Ch 4", "Ch 5", "Ch 6", "Ch 7", "Ch 8", "Ch 9", "Ch 10", "Ch 11", "Ch 12", "Ch 13", "Ch 14", "Ch 15", "Ch 16", "Ch 17", "Ch 18", "Ch 19", "Ch 20", "", "Ch 22", "Ch 23", "Ch 24", "Ch 25", "Ch 26", "Ch 27", "Ch 28", "Ch 29", "Ch 30", "Ch 31", "Paired", "Unpaired"}, "SG Pair Ch 22":enum16{"Ch 0", "Ch 1", "Ch 2", "Ch 3", "Ch 4", "Ch 5", "Ch 6", "Ch 7", "Ch 8", "Ch 9", "Ch 10", "Ch 11", "Ch 12", "Ch 13", "Ch 14", "Ch 15", "Ch 16", "Ch 17", "Ch 18", "Ch 19", "Ch 20", "Ch 21", "", "Ch 23", "Ch 24", "Ch 25", "Ch 26", "Ch 27", "Ch 28", "Ch 29", "Ch 30", "Ch 31", "Paired", "Unpaired"}, "SG Pair Ch 23":enum16{"Ch 0", "Ch 1", "Ch 2", "Ch 3", "Ch 4", "Ch 5", "Ch 6", "Ch 7", "Ch 8", "Ch 9", "Ch 10", "Ch 11", "Ch 12", "Ch 13", "Ch 14", "Ch 15", "Ch 16", "Ch 17", "Ch 18", "Ch 19", "Ch 20", "Ch 21", "Ch 22", "", "Ch 24", "Ch 25", "Ch 26", "Ch 27", "Ch 28", "Ch 29", "Ch 30", "Ch 31", "Paired", "Unpaired"}, "SG Pair Ch 24":enum16{"Ch 0", "Ch 1", "Ch 2", "Ch 3", "Ch 4", "Ch 5", "Ch 6", "Ch 7", "Ch 8", "Ch 9", "Ch 10", "Ch 11", "Ch 12", "Ch 13", "Ch 14", "Ch 15", "Ch 16", "Ch 17", "Ch 18", "Ch 19", "Ch 20", "Ch 21", "Ch 22", "Ch 23", "", "Ch 25", "Ch 26", "Ch 27", "Ch 28", "Ch 29", "Ch 30", "Ch 31", "Paired", "Unpaired"}, "SG Pair Ch 25":enum16{"Ch 0", "Ch 1", "Ch 2", "Ch 3", "Ch 4", "Ch 5", "Ch 6", "Ch 7", "Ch 8", "Ch 9", "Ch 10", "Ch 11", "Ch 12", "Ch 13", "Ch 14", "Ch 15", "Ch 16", "Ch 17", "Ch 18", "Ch 19", "Ch 20", "Ch 21", "Ch 22", "Ch 23", "Ch 24", "", "Ch 26", "Ch 27", "Ch 28", "Ch 29", "Ch 30", "Ch 31", "Paired", "Unpaired"}, "SG Pair Ch 26":enum16{"Ch 0", "Ch 1", "Ch 2", "Ch 3", "Ch 4", "Ch 5", "Ch 6", "Ch 7", "Ch 8", "Ch 9", "Ch 10", "Ch 11", "Ch 12", "Ch 13", "Ch 14", "Ch 15", "Ch 16", "Ch 17", "Ch 18", "Ch 19", "Ch 20", "Ch 21", "Ch 22", "Ch 23", "Ch 24", "Ch 25", "", "Ch 27", "Ch 28", "Ch 29", "Ch 30", "Ch 31", "Paired", "Unpaired"}, "SG Pair Ch 27":enum16{"Ch 0", "Ch 1", "Ch 2", "Ch 3", "Ch 4", "Ch 5", "Ch 6", "Ch 7", "Ch 8", "Ch 9", "Ch 10", "Ch 11", "Ch 12", "Ch 13", "Ch 14", "Ch 15", "Ch 16", "Ch 17", "Ch 18", "Ch 19", "Ch 20", "Ch 21", "Ch 22", "Ch 23", "Ch 24", "Ch 25", "Ch 26", "", "Ch 28", "Ch 29", "Ch 30", "Ch 31", "Paired", "Unpaired"}, "SG Pair Ch 28":enum16{"Ch 0", "Ch 1", "Ch 2", "Ch 3", "Ch 4", "Ch 5", "Ch 6", "Ch 7", "Ch 8", "Ch 9", "Ch 10", "Ch 11", "Ch 12", "Ch 13", "Ch 14", "Ch 15", "Ch 16", "Ch 17", "Ch 18", "Ch 19", "Ch 20", "Ch 21", "Ch 22", "Ch 23", "Ch 24", "Ch 25", "Ch 26", "Ch 27", "", "Ch 29", "Ch 30", "Ch 31", "Paired", "Unpaired"}, "SG Pair Ch 29":enum16{"Ch 0", "Ch 1", "Ch 2", "Ch 3", "Ch 4", "Ch 5", "Ch 6", "Ch 7", "Ch 8", "Ch 9", "Ch 10", "Ch 11", "Ch 12", "Ch 13", "Ch 14", "Ch 15", "Ch 16", "Ch 17", "Ch 18", "Ch 19", "Ch 20", "Ch 21", "Ch 22", "Ch 23", "Ch 24", "Ch 25", "Ch 26", "Ch 27", "Ch 28", "", "Ch 30", "Ch 31", "Paired", "Unpaired"}, "SG Pair Ch 30":enum16{"Ch 0", "Ch 1", "Ch 2", "Ch 3", "Ch 4", "Ch 5", "Ch 6", "Ch 7", "Ch 8", "Ch 9", "Ch 10", "Ch 11", "Ch 12", "Ch 13", "Ch 14", "Ch 15", "Ch 16", "Ch 17", "Ch 18", "Ch 19", "Ch 20", "Ch 21", "Ch 22", "Ch 23", "Ch 24", "Ch 25", "Ch 26", "Ch 27", "Ch 28", "Ch 29", "", "Ch 31", "Paired", "Unpaired"}, "SG Pair Ch 31":enum16{"Ch 0", "Ch 1", "Ch 2", "Ch 3", "Ch 4", "Ch 5", "Ch 6", "Ch 7", "Ch 8", "Ch 9", "Ch 10", "Ch 11", "Ch 12", "Ch 13", "Ch 14", "Ch 15", "Ch 16", "Ch 17", "Ch 18", "Ch 19", "Ch 20", "Ch 21", "Ch 22", "Ch 23", "Ch 24", "Ch 25", "Ch 26", "Ch 27", "Ch 28", "Ch 29", "Ch 30", "", "Paired", "Unpaired"}}, cluster{"PF Condition 0":bool, "PF Condition 1":bool, "PF Condition 2":bool, "PF Condition 3":bool, "PF Condition 4":bool, "PF Condition 5":bool, "PF Condition 6":bool, "PF Condition 7":bool, "PF Condition 8":bool, "PF Condition 9":bool, "PF Condition 10":bool, "PF Condition 11":bool, "PF Condition 12":bool, "PF Condition 13":bool, "PF Condition 14":bool, "PF Condition 15":bool, "PF Condition 16":bool, "PF Condition 17":bool, "PF Condition 18":bool, "PF Condition 19":bool, "PF Condition 20":bool, "PF Condition 21":bool, "PF Condition 22":bool, "PF Condition 23":bool, "PF Condition 24":bool, "PF Condition 25":bool, "PF Condition 26":bool, "PF Condition 27":bool, "PF Condition 28":bool, "PF Condition 29":bool, "PF Condition 30":bool, "PF Condition 31":bool}, cluster{"PF Info":string, "PF Info":string, "PF Info":string, "PF Info":string, "PF Info":string, "PF Info":string, "PF Info":string, "PF Info":string, "PF Info":string, "PF Info":string, "PF Info":string, "PF Info":string, "PF Info":string, "PF Info":string, "PF Info":string, "PF Info":string, "PF Info":string, "PF Info":string, "PF Info":string, "PF Info":string, "PF Info":string, "PF Info":string, "PF Info":string, "PF Info":string, "PF Info":string, "PF Info":string, "PF Info":string, "PF Info":string, "PF Info":string, "PF Info":string, "PF Info":string, "PF Info":string}}, "Value":cluster{"Programmer Info":string, "Value":dbl, "Value":dbl}}
  T57 = cluster{"Samples per test (Sa)":i32, "Sample Rate (Sa/sec)":dbl, "Trigger Slope":i32, "Trigger Level (V)":dbl, "Pre-Trigger (%)":i32}
  T58 = typedef "DialogType.ctl" = u16
  T59 = cluster{bool, "Enable Ch 1":bool, "Enable Ch 2":bool, "Enable Ch 3":bool, "Enable Ch 4":bool, "Enable Ch 5":bool, "Enable Ch 6":bool, "Enable Ch 7":bool, "Enable Ch 8":bool, "Enable Ch 9":bool, "Enable Ch 10":bool, "Enable Ch 11":bool, "Enable Ch 12":bool, "Enable Ch 13":bool, "Enable Ch 14":bool, "Enable Ch 15":bool, "Enable Ch 16":bool, "Enable Ch 17":bool, "Enable Ch 18":bool, "Enable Ch 19":bool, "Enable Ch 20":bool, "Enable Ch 21":bool, "Enable Ch 22":bool, "Enable Ch 23":bool, "Enable Ch 24":bool, "Enable Ch 25":bool, "Enable Ch 26":bool, "Enable Ch 27":bool, "Enable Ch 28":bool, "Enable Ch 29":bool, "Enable Ch 30":bool, "Enable Ch 31":bool}
  T60 = cluster{"Name (Laser Gate)":string, "Name Ch 1":string, "Name Ch 2":string, "Name Ch 3":string, "Name Ch 4":string, "Name Ch 5":string, "Name Ch 6":string, "Name Ch 7":string, "Name Ch 8":string, "Name Ch 9":string, "Name Ch 10":string, "Name Ch 11":string, "Name Ch 12":string, "Name Ch 13":string, "Name Ch 14":string, "Name Ch 15":string, "Name Ch 16":string, "Name Ch 17":string, "Name Ch 18":string, "Name Ch 19":string, "Name Ch 20":string, "Name Ch 21":string, "Name Ch 22":string, "Name Ch 23":string, "Name Ch 24":string, "Name Ch 25":string, "Name Ch 26":string, "Name Ch 27":string, "Name Ch 28":string, "Name Ch 29":string, "Name Ch 30":string, "Name Ch 31":string}
  T61 = cluster{"Voltage Max Ch 0":dbl, "Voltage Max Ch 1":dbl, "Voltage Max Ch 2":dbl, "Voltage Max Ch 3":dbl, "Voltage Max Ch 4":dbl, "Voltage Max Ch 5":dbl, "Voltage Max  Ch 6":dbl, "Voltage Max Ch 7":dbl, "Voltage Max Ch 8":dbl, "Voltage Max Ch 9":dbl, "Voltage Max Ch 10":dbl, "Voltage Max Ch 11":dbl, "Voltage Max Ch 12":dbl, "Voltage Max Ch 13":dbl, "Voltage Max Ch 14":dbl, "Voltage Max Ch 15":dbl, "Voltage Max Ch 16":dbl, "Voltage Max Ch 17":dbl, "Voltage Max Ch 18":dbl, "Voltage Max Ch 19":dbl, "Voltage Max Ch 20":dbl, "Voltage Max Ch 21":dbl, "Voltage Max Ch 22":dbl, "Voltage Max Ch 23":dbl, "Voltage Max Ch 24":dbl, "Voltage Max Ch 25":dbl, "Voltage Max Ch 26":dbl, "Voltage Max Ch 27":dbl, "Voltage Max Ch 28":dbl, "Voltage Max Ch 29":dbl, "Voltage Max Ch 30":dbl, "Voltage Max Ch 31":dbl}
  T62 = cluster{"Voltage Min Ch 0":dbl, "Voltage Min Ch 1":dbl, "Voltage Min Ch 2":dbl, "Voltage Min Ch 3":dbl, "Voltage Min Ch 4":dbl, "Voltage Min Ch 5":dbl, "Voltage Min Ch 6":dbl, "Voltage Min Ch 7":dbl, "Voltage Min Ch 8":dbl, "Voltage Min Ch 9":dbl, "Voltage Min Ch 10":dbl, "Voltage Min Ch 11":dbl, "Voltage Min Ch 12":dbl, "Voltage Min Ch 13":dbl, "Voltage Min Ch 14":dbl, "Voltage Min Ch 15":dbl, "Voltage Min Ch 16":dbl, "Voltage Min Ch 17":dbl, "Voltage Min Ch 18":dbl, "Voltage Min Ch 19":dbl, "Voltage Min Ch 20":dbl, "Voltage Min Ch 21":dbl, "Voltage Min Ch 22":dbl, "Voltage Min Ch 23":dbl, "Voltage Min Ch 24":dbl, "Voltage Min Ch 25":dbl, "Voltage Min Ch 26":dbl, "Voltage Min Ch 27":dbl, "Voltage Min Ch 28":dbl, "Voltage Min Ch 29":dbl, "Voltage Min Ch 30":dbl, "Voltage Min Ch 31":dbl}
  T63 = cluster{"PF Info":string, "PF Info":string, "PF Info":string, "PF Info":string, "PF Info":string, "PF Info":string, "PF Info":string, "PF Info":string, "PF Info":string, "PF Info":string, "PF Info":string, "PF Info":string, "PF Info":string, "PF Info":string, "PF Info":string, "PF Info":string, "PF Info":string, "PF Info":string, "PF Info":string, "PF Info":string, "PF Info":string, "PF Info":string, "PF Info":string, "PF Info":string, "PF Info":string, "PF Info":string, "PF Info":string, "PF Info":string, "PF Info":string, "PF Info":string, "PF Info":string, "PF Info":string}
  T64 = cluster{"Physical Channels Ch 0":tag, "Physical Channel Ch 1":tag, "Physical Channel Ch 2":tag, "Physical Channels Ch 3":tag, "Physical Channel Ch 4":tag, "Physical Channel Ch 5":tag, "Physical Channels Ch 6":tag, "Physical Channel Ch 7":tag, "Physical Channel Ch 8":tag, "Physical Channel Ch 9":tag, "Physical Channel Ch 10":tag, "Physical Channel Ch 11":tag, "Physical Channel Ch 12":tag, "Physical Channel Ch 13":tag, "Physical Channel Ch 14":tag, "Physical Channel Ch 15":tag, "Physical Channel Ch 16":tag, "Physical Channel Ch 17":tag, "Physical Channel Ch 18":tag, "Physical Channel Ch 19":tag, "Physical Channel Ch 20":tag, "Physical Channel Ch 21":tag, "Physical Channel Ch 22":tag, "Physical Channel Ch 23":tag, "Physical Channel Ch 24":tag, "Physical Channel Ch 25":tag, "Physical Channel Ch 26":tag, "Physical Channel Ch 27":tag, "Physical Channel Ch 28":tag, "Physical Channel Ch 29":tag, "Physical Channel Ch 30":tag, "Physical Channel Ch 31":tag}
diagram:
  # "1) Fix Velocity and Acceleration ? - Diagnose to see if still a problem"
  # "To - Do \n1) Pair Strain Channels for Long and Bend Seperation - Done\n2) Strain Rate Cal - Done\n3) Vel 2 Accel Calc - Done\n4) Saving Data File - Done\n5) Create State Machine - Done\n6) In Idle Stage - Update/Tie interface actions to turn things on/off - Done"
  # "Add Strain Sep Name? - no for now, use first 5 characters of SG name"
  # "To do: Finish State machine\n- tie paired stain channels together - Done\n- finish GUI enable/disable of other channels - Done\n- Create load data function - Done\n - create save data functions for rate and seperated data - Done"
  # "32 Channel Shock and Dyanmics Lab Code - Hopkinson Bar\nWritten By: Jacob Dodson\nRevisions By: Mitzi Dennis\n\nRev: 3.0\nDate: August 3, 2016\n\nUpdates:\n - added 16 channels (now have 32)\n - added continuous feature (allows continuous sampling of data at lower sampling rate)\n     - includes continuous/updated readout on graph during test\n - added active tab functions\n - updated velocity of striker measurement (different laser setup)\n\n\nEventually:\n - add automation of PF information into channel settings"
  n1 = while {
    shift-right: [w9] -> _
    shift-left: 32CHDAQ_-_Cases."Initialize" ("Program State") -> [w6]
    shift-right: [w8] -> _
    shift-left: errorcluster {"status"=FALSE, "code"=0, "source"=""} ("error out") -> [w7]
    stop <- w10 stop-if-true
    n2 = flat-sequence {
      tunnel: w7 -> [w12]
      tunnel: w6 -> [w11]
      tunnel: [w14] -> w5
      tunnel: [w13] -> w4
      tunnel: [w3266] -> w8
      tunnel: [w3267] -> w9
      tunnel: w5 -> [w3267]
      tunnel: w4 -> [w3266]
      frame #0 {
        (unwired) 32CHDAQ_-_Cases."Initialize" ("Program State")
        n3 = case shown="\"Execute\"" w11 {
          tunnel: [w18 w32 w2274 w2468 w2538 w2704 w2758] -> w13
          tunnel: [32CHDAQ_-_Cases."Idle" ("Program State") w35 w2283 w2491 32CHDAQ_-_Cases."Idle" ("Program State") w2702 32CHDAQ_-_Cases."End" ("Program State")] -> w14
          tunnel: w12 -> [w20 w34 w2276 w2421 _ w2704 w2766]
          frame "Initialize", Default {
            w16 = FALSE ("Finished Saving Data")
            w25 = waveform(dbl)[] [] ("array")
            # "Reset Buttons"
            # "Clear Graphs"
            n4 = control-ref of="This VI"() -> ()  [unwired: 1 out]
            n5 = property on="Bending Strain" class="WFGraph (strict)"(error in=w20, "Value"=w25) -> (error out=w30:errorcluster)  [unwired: 1 in, 1 out]
            n6 = property on="Longitudinal Strain" class="WFGraph (strict)"(error in=w30, "Value"=w25) -> (error out=w29:errorcluster)  [unwired: 1 in, 1 out]
            n7 = property on="Raw Data" class="WFGraph (strict)"(error in=w29, "Value"=w25) -> (error out=w28:errorcluster)  [unwired: 1 in, 1 out]
